vi "Cannon Process.vi"(0 "error in":errorcluster) -> ()   [LabVIEW 2013]
uses:
  Cannon Global Data.vi
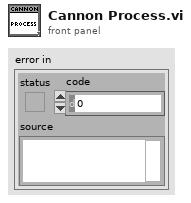
[diagram p1: front panel]
types:
  T1 = typedef "WPI_SolenoidValue.ctl" = enum16{"Off", "On", "Forward", "Reverse"}
  T2 = cluster{"Motor":dbl, "Solenoid":T1, "BallInMS":bool, "ClutchMS":bool, "Potentiometer":dbl}
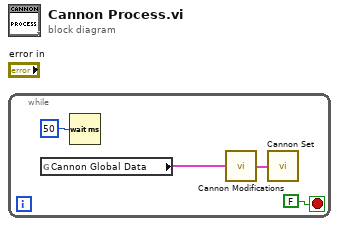
[diagram p0: block diagram]
diagram:
  n1 = while {
    stop <- FALSE stop-if-true
    n2 = global read "Cannon Global Data.vi" "Cannon Global Data"() -> (w1:T2)
    n3 = Wait (ms)(milliseconds to wait=u32 50) -> ()  [unwired: 1 out]
    n4 = call "Cannon Modifications.vi"("Cannon Global Data In"=w1) -> ("Cannon Global Data Out"=w2:T2)
    n5 = call "Cannon Set.vi"("Cannon Global Data"=w2) -> ()
  }
